vi "lsl push sample buf.vi"(8 "error in (no error)":errorcluster, 9 "lengths":u32, 10 "data":string, 11 "outlet":T1) -> (0 "error out":errorcluster, 2 "function return":i32)   [LabVIEW 2016, in "Lab Streaming Layer.lvlib"]
doc: "extern LIBLSL_C_API int32_t lsl_push_sample_buf(lsl_outlet out, const char **data, const uint32_t *lengths);"
uses:
  Lab Streaming Layer.lvlib
  liblsl-LabVIEW-master/liblsl-LabVIEW-master/lsl.dll
  Custom Controls/lsl_outlet.ctl
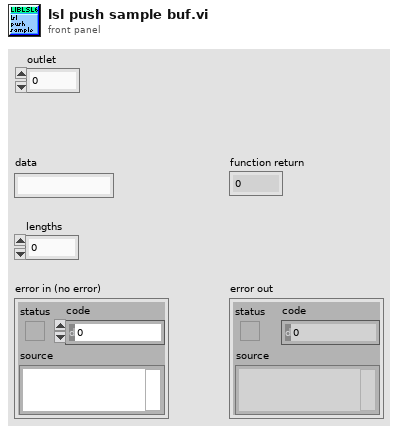
[diagram p1: front panel]
types:
  T1 = typedef "liblsl-LabVIEW.lvlib/lsl_outlet.ctl" = u64
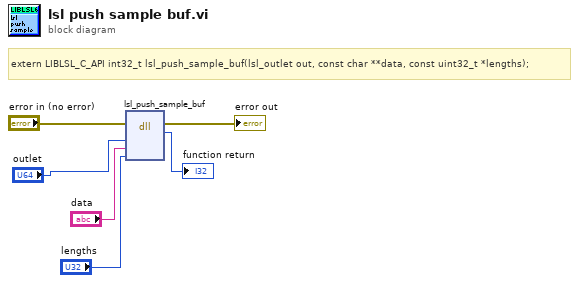
[diagram p0: block diagram]
diagram:
  # "extern LIBLSL_C_API int32_t lsl_push_sample_buf(lsl_outlet out, const char **data, const uint32_t *lengths);"
  n1 = dll-call lib="E:/LabStreamingLayer/liblsl-LabVIEW-master/liblsl-LabVIEW-master/lsl.dll" fn="lsl_push_sample_buf"(error in="error in (no error)", "out"="outlet", "data"="data", "lengths"="lengths") -> (error out=→"error out":errorcluster, "return type"=→"function return":i32)  [unwired: 5 in, 1 out]
